vi "TIME_TO_MINUTES.vi"(10 "START TIME":timestamp=timestamp(3597615000 s since 1904-01-01) format="%<%H:%M:%S>T", 11 "END TIME":timestamp=timestamp(3597643859 s since 1904-01-01) format="%<%H:%M:%S>T") -> (3 "In Minutes":i32)   [LabVIEW 2017]
panel:
  out "substring 3":string
  out "substring 2":string
  out "substring":string
  out "resulting string":string
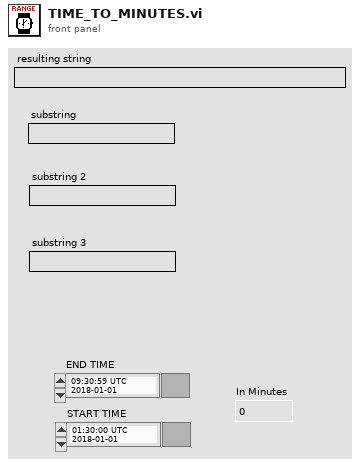
[diagram p1: front panel]
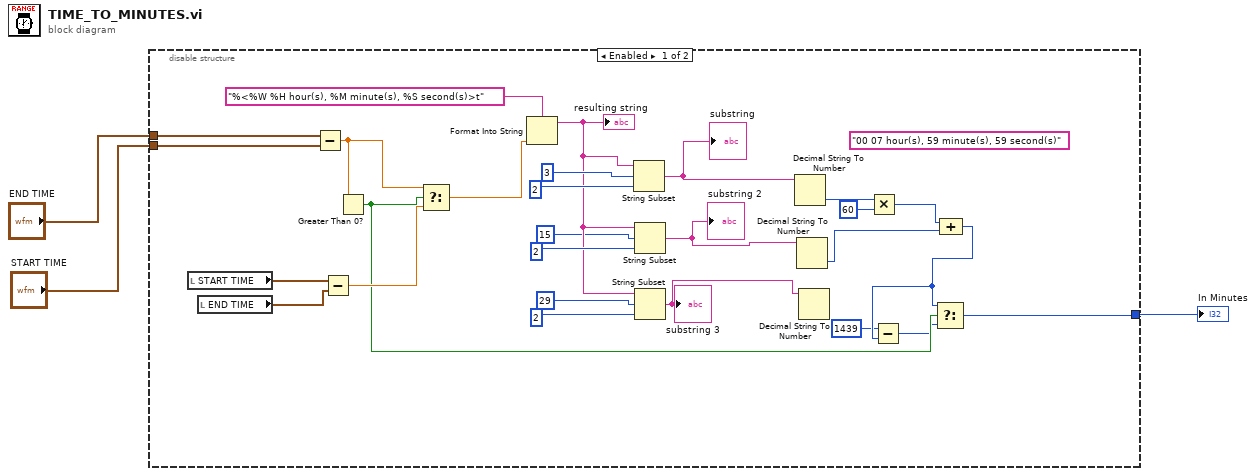
[diagram p0: block diagram]
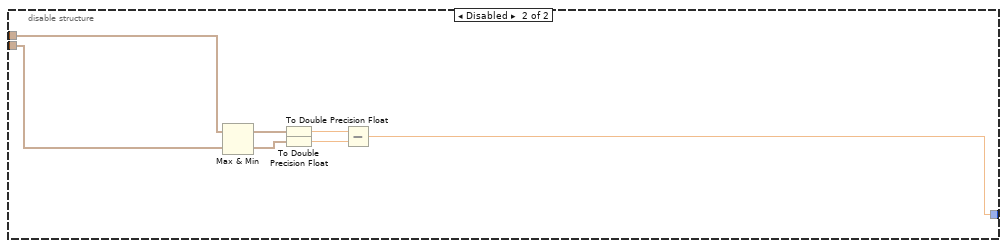
[diagram p2: hidden frame]
diagram:
  n1 = disable-structure shown="Enabled" {
    disable-tunnel: "END TIME" -> [w29 w33]
    disable-tunnel: "START TIME" -> [w28 w32]
    disable-tunnel: [w7 w31] -> w1
    frame Enabled {
      (unwired) "00 07 hour(s), 59 minute(s), 59 second(s)" ("resulting string")
      n2 = local read "START TIME"() -> (w12:timestamp)
      n3 = local read "END TIME"() -> (w11:timestamp)
      n4 = Subtract(x=w29, y=w28) -> (x-y=w13:dbl)
      n5 = Subtract(x=w12, y=w11) -> (x-y=w10:dbl)
      n6 = Greater Than 0?(x=w13) -> (x > 0?=w8:bool)
      n7 = Select(t=w13, s=w8, f=w10) -> (s? t:f=w9:dbl)
      n8 = Format Into String(format string="%<%W %H hour(s), %M minute(s), %S second(s)>t", w9) -> (resulting string=w23:string)  [unwired: 2 in, 1 out]
      "resulting string" <- w23
      n9 = String Subset(string=w23, offset (0)=3, length (rest)=2 ("offset (0)")) -> (substring=w20:string)
      "substring" <- w20
      n10 = String Subset(string=w23, offset (0)=15, length (rest)=2 ("offset (0)")) -> (substring=w19:string)
      "substring 2" <- w19
      n11 = String Subset(string=w23, offset (0)=29, length (rest)=2 ("offset (0)")) -> (substring=w18:string)
      "substring 3" <- w18
      n12 = Decimal String To Number(string=w20) -> (number=w17:i32)  [unwired: 2 in, 1 out]
      n13 = Decimal String To Number(string=w19) -> (number=w14:i32)  [unwired: 2 in, 1 out]
      n14 = Decimal String To Number(string=w18) -> ()  [unwired: 2 in, 2 out]
      n15 = Multiply(x=w17, y=60) -> (x*y=w15:i32)
      n16 = Compound Arithmetic op=ADD(w15, w14) -> (w6:i32)
      n17 = Subtract(x=1439, y=w6) -> (x-y=w4:i32)
      n18 = Select(t=w6, s=w8, f=w4) -> (s? t:f=w7:i32)
    }
    frame Disabled {
      n19 = Max & Min(x=w33, y=w32) -> (max(x,y)=w37:timestamp, min(x,y)=w36:timestamp)
      n20 = To Double Precision Float(number=w37) -> (double precision float=w35:dbl)
      n21 = To Double Precision Float(number=w36) -> (double precision float=w34:dbl)
      n22 = Subtract(x=w35, y=w34) -> (x-y=w31:dbl)
    }
  }
  "In Minutes" <- w1
